vi "Measure.vi"(8 "error in (no error)":errorcluster, 10 "unit":T1, 11 "controller in":refnum<class "Temperature Controller.lvclass">) -> (0 "error out":errorcluster, 2 "measurement":dbl, 3 "controller out":refnum<class "Temperature Controller.lvclass">)   [LabVIEW 2019, in "Temperature Controller.lvclass"]
uses:
  Temperature Controller.lvclass
  Units.ctl
  Temperature Controller.lvclass/Temperature Controller.ctl
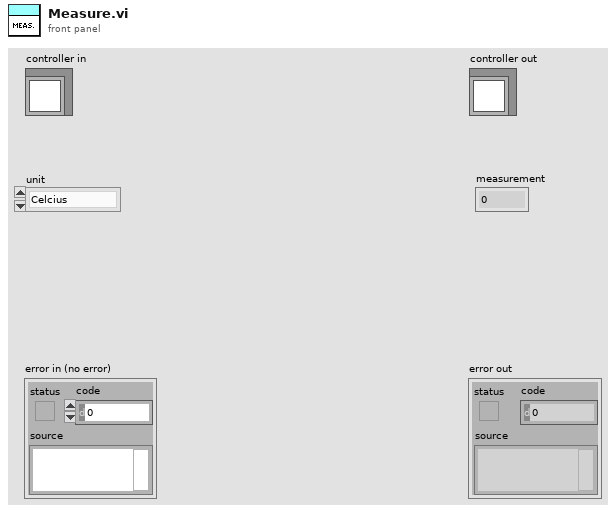
[diagram p1: front panel]
types:
  T1 = typedef "Temperature Controller.lvclass/Units.ctl" = enum16{"Celcius", "Fahrenheit"}
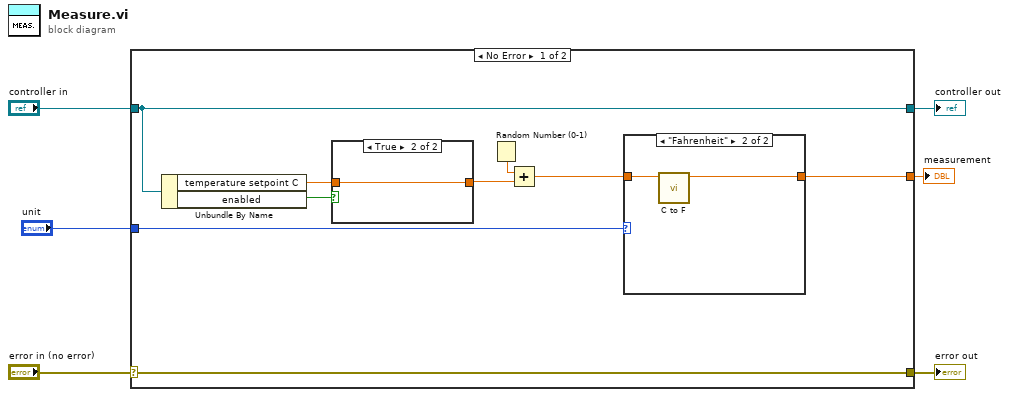
[diagram p0: block diagram]
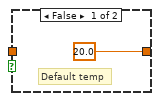
[diagram p2: hidden frame]
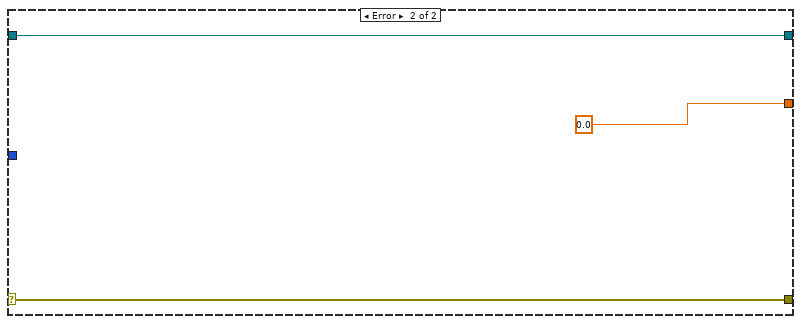
[diagram p4: hidden frame]
diagram:
  n1 = case shown="No Error" "error in (no error)" {
    selector: "error in (no error)" -> [w15 w23]
    tunnel: [w15 w23] -> w5
    tunnel: [w10 w22] -> w3
    tunnel: "controller in" -> [w10 w22]
    tunnel: "unit" -> [w13 _]
    tunnel: [w11 0.0] -> w1
    frame No Error {
      n2 = Unbundle By Name(w10) -> ("temperature setpoint C"=w8:dbl, "enabled"=w9:bool)
      n3 = case shown="True" w9 {
        tunnel: w8 -> [_ w17]
        tunnel: [20.0 ("temperature setpoint C") w17] -> w7
        frame False {
          # "Default temp"
        }
        frame True {
        }
      }
      n4 = Random Number (0-1)() -> (number: 0 to 1=w14:dbl)
      n5 = Add(x=w14, y=w7) -> (x+y=w12:dbl)
      n6 = case shown="\"Fahrenheit\"" w13 {
        tunnel: w12 -> [w18 w20]
        tunnel: [w18 w19] -> w11
        frame "Celcius", Default {
        }
        frame "Fahrenheit" {
          n7 = call "C to F.vi"("celsius"=w20) -> ("fahrenheit"=w19:dbl)  [unwired: 10 in]
        }
      }
    }
    frame Error {
    }
  }
  "error out" <- w5
  "controller out" <- w3
  "measurement" <- w1
